vi "SeCrTs-Obtain Message Queue_R.vi"(7 "max queue size (-1, unlimited)":i32=10, 8 "error in (no error)":errorcluster) -> (0 "error out":errorcluster, 1 "queue out":refnum<queue>, 3 "Message Queue":refnum<queue>)   [LabVIEW 2022 SP3]
uses:
  RT Controls/SeCrTs-Message Cluster_R.ctl
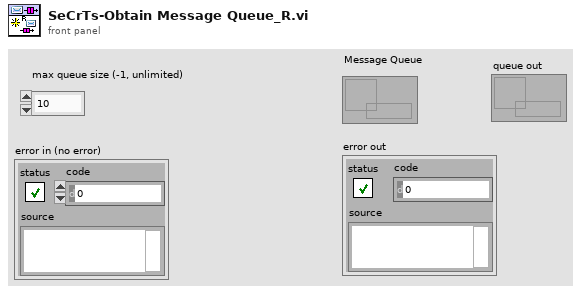
[diagram p1: front panel]
types:
  T1 = cluster{"Error Code":string, "Error Source":string}
  T2 = typedef "SeCrTs-Message Cluster_R.ctl" = cluster{"Message":string, "Message Data":variant}
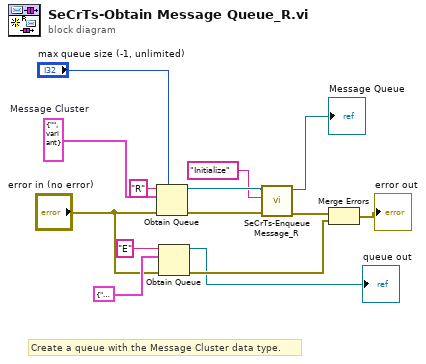
[diagram p0: block diagram]
diagram:
  w14 = T2 {"Message"="", "Message Data"=variant}  # Message Cluster
  # "Create a queue with the Message Cluster data type."
  n1 = Obtain Queue(max queue size (-1, unlimited)="max queue size (-1, unlimited)", name (unnamed)="R", element data type=w14, error in (no error)="error in (no error)") -> (queue out=w3:refnum<queue>, error out=w5:errorcluster)  [unwired: 1 in, 1 out]
  n2 = Obtain Queue(name (unnamed)="E", element data type=T1 {"Error Code"="", "Error Source"=""} ("element"), error in (no error)="error in (no error)") -> (queue out=→"queue out":refnum<queue>, error out=w7:errorcluster)  [unwired: 2 in, 1 out]
  n3 = call "SeCrTs-Enqueue Message_R.vi"("error in (no error)"=w5, "Message"="Initialize", "Message Queue"=w3) -> ("error out"=w4:errorcluster, "dup Message Queue"=→"Message Queue":refnum<queue>)  [unwired: 7 in]
  n4 = Merge Errors(w4, w7) -> (→"error out":errorcluster)
